vi "PositionToDuty.vi"(6 "lower limit":dbl, 7 "upper limit":dbl, 9 "freq [Hz] in":dbl=50.0, 10 "null offset in":bool, 11 "Posición":dbl) -> (1 "duty cycle [%] 2":dbl, 2 "pulse width [ms] 2":dbl=1.5, 3 "offset [%FS] 2":dbl, 4 "DutyCycle":dbl, 5 "Grados":dbl(graph))   [LabVIEW 2014]
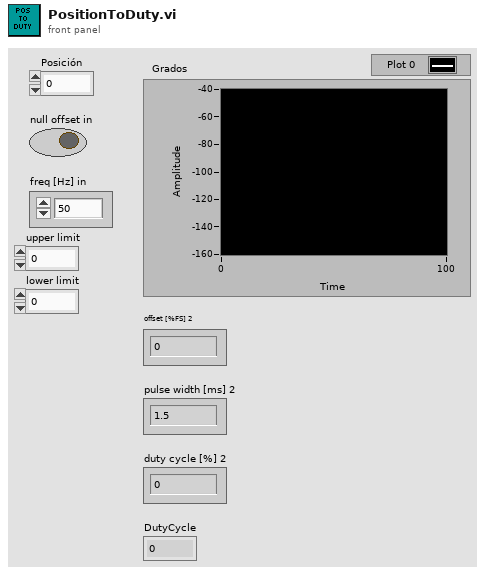
[diagram p1: front panel]
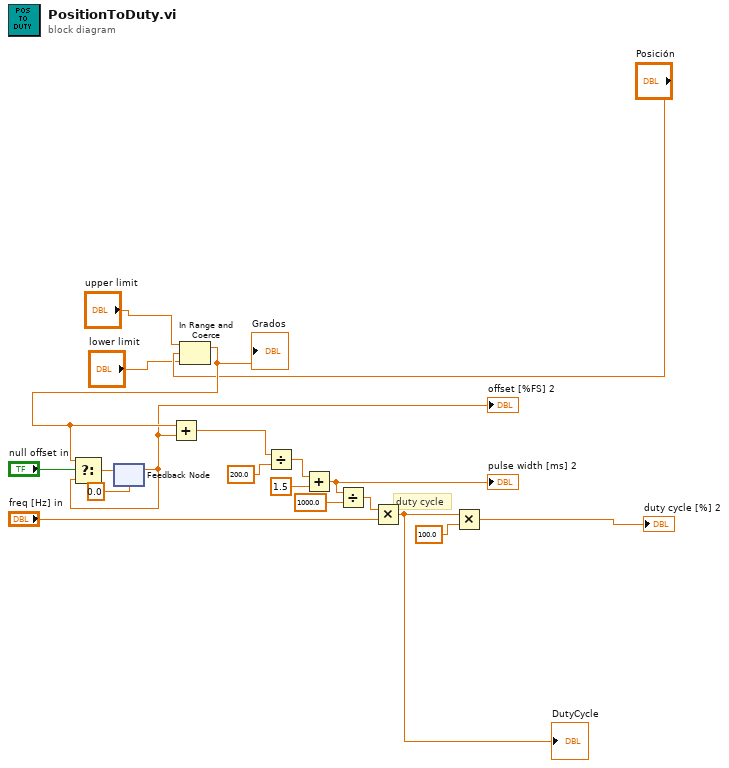
[diagram p0: block diagram]
diagram:
  # "duty cycle"
  n1 = feedback #1(0.0 ("position [%FS]")) -> (w9:dbl)
  "offset [%FS] 2" <- w9
  n2 = In Range and Coerce(upper limit="upper limit", x="Posición", lower limit="lower limit") -> (coerced(x)=w19:dbl)  [unwired: 1 out]
  "Grados" <- w19
  n3 = Select(t=w19, s="null offset in", f=w9) -> (s? t:f=w8:dbl)
  n4 = feedback-in #1(w8) -> ()
  n5 = Add(x=w19, y=w9) -> (x+y=w13:dbl)
  n6 = Divide(x=w13, y=200.0) -> (x/y=w3:dbl)
  n7 = Add(x=w3, y=1.5) -> (x+y=w5:dbl)
  "pulse width [ms] 2" <- w5
  n8 = Divide(x=w5, y=1000.0) -> (x/y=w10:dbl)
  n9 = Multiply(x=w10, y="freq [Hz] in") -> (x*y=w18:dbl)
  "DutyCycle" <- w18
  n10 = Multiply(x=w18, y=100.0) -> (x*y=→"duty cycle [%] 2":dbl)
